vi "Process-error-general.vi"(8 "error in (no error)":errorcluster, 11 "Errors in":T1) -> (0 "error out":errorcluster, 3 "Errors out":T1)   [LabVIEW 2013, in "Error-handling.lvlib" / "Errors.lvclass"]
uses:
  Errors.lvclass
  Object-reference.ctl
  Errors.lvclass/Errors.ctl
  Read Display error dialog.vi
  Read Language.vi
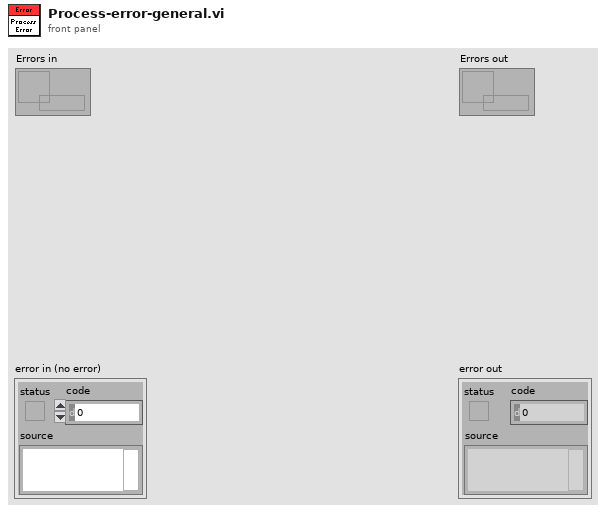
[diagram p1: front panel]
types:
  T1 = typedef "Error-handling.lvlib/Errors.lvclass/Object-reference.ctl" = refnum<data-value>
  T2 = typedef "Error-handling.lvlib/Errors.lvclass/Languages.ctl" = enum16{"English"}
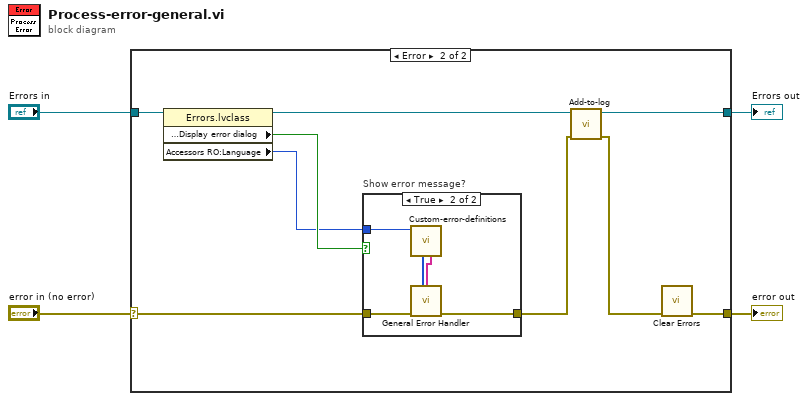
[diagram p0: block diagram]
diagram:
  n1 = case shown="Error" "error in (no error)" {
    selector: "error in (no error)" -> [w5 w15]
    tunnel: [w5 w8] -> w3
    tunnel: [w6 w14] -> w1
    tunnel: "Errors in" -> [w6 w11]
    frame No Error {
    }
    frame Error {
      n2 = property class="Errors.lvclass"(reference=w11) -> (reference out=w10:T1, "Accessors RO:Display error dialog"=w9:bool, "Accessors RO:Language"=w7:T2)  [unwired: 1 in, 1 out]
      n3 = case "Show error message?" shown="True" w9 {
        tunnel: w15 -> [w16 w21]
        tunnel: [w16 w20] -> w12
        tunnel: w7 -> [_ w17]
        frame False {
        }
        frame True {
          n4 = call "Custom-error-definitions.vi"("Language"=w17) -> ("Descriptions"=w18:string[], "Error codes"=w19:i32[])  [unwired: 8 in, 1 out]
          n5 = call <vilib>:"General Error Handler.vi"("[user-defined codes]"=w19, "[user-defined descriptions]"=w18, "error in (no error)"=w21) -> ("error out"=w20:errorcluster)  [unwired: 8 in, 4 out]
        }
      }
      n6 = call "Add-to-log.vi"("error in (no error)"=w12, "Errors in"=w10) -> ("error out"=w13:errorcluster, "Errors out"=w14:T1)  [unwired: 8 in]
      n7 = call <vilib>:"Clear Errors.vi"("error in (no error)"=w13) -> ("error out"=w8:errorcluster)  [unwired: 6 in]
    }
  }
  "error out" <- w3
  "Errors out" <- w1
